vi "REQ full lifecycle.vi"(0 "endpoint":string="tcp://127.0.0.1:5555", 1 "Julia user functions script":path=path "dummy.jl", 2 "LV Client state in":T2, 5 "data to send":string="hello", 7 "ZMQ new Timeouts in":T1={"SNDTIMEO"=-1, "RCVTIMEO"=-1}, 9 "Force command":bool, 11 "error in":errorcluster, 12 "command":T3, 13 "Jl Server state in":T2) -> (3 "LV Client state out":T2, 4 "server response":string, 6 "socket out":refnum<class "zmq_socket.lvclass">, 8 "ZMQ timeouts out":cluster{"previous":T1, "current":T1}={"previous"={"SNDTIMEO"=-1, "RCVTIMEO"=-1}, "current"={"SNDTIMEO"=-1, "RCVTIMEO"=-1}}, 10 "timeout?":bool, 14 "Jl Server state out":T2, 15 "error out":errorcluster)   [LabVIEW 2018, in "LV-0mq-Julia_roundtrip-lib.lvlib"]
uses:
  LV-0mq-Julia_roundtrip-lib.lvlib
  Commands.ctl
  Server or client state.ctl
  ZMQ timeouts.ctl
  <vilib>/addons/zeromq/zmq_socket.lvclass
  <vilib>/addons/zeromq/zmq_context.lvclass
  commands LV2Jl.ctl
  expected server response.ctl
  <vilib>/addons/zeromq/socket_options.ctl
  <vilib>/Utility/error.llb/Error Cluster From Error Code.vi
  ZMQ timeouts global.vi
  <vilib>/addons/zeromq/zmq_getsocketopt_int.vi
  <vilib>/ErrorRing/Error Ring.xnode
  <vilib>/addons/zeromq/zeromq.lvlib
panel:
  out "return code":i32
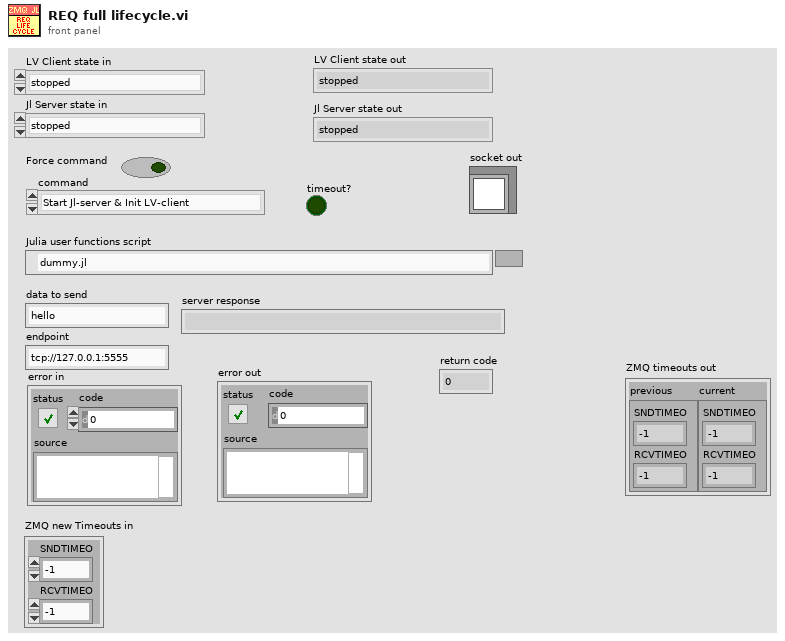
[diagram p1: front panel]
types:
  T1 = typedef "LV-0mq-Julia_roundtrip-lib.lvlib/ZMQ timeouts.ctl" = cluster{"SNDTIMEO":i32, "RCVTIMEO":i32}
  T2 = typedef "LV-0mq-Julia_roundtrip-lib.lvlib/Server or client state.ctl" = enum16{"stopped", "running", "unknown"}
  T3 = typedef "LV-0mq-Julia_roundtrip-lib.lvlib/Commands.ctl" = enum16{"Start Jl-server & Init LV-client", "Send request & Get response ", "Stop Jl-server & Cleanup LV-client", "Cleanup LV-client", "Start Jl-server", "Stop Jl-server", "Init LV-Client", "Cleanup LV-Client", "(not allowed)", "Set LV Client state", "Set Jl Server state", "set ZMQ timeout", "read ZMQ timeout", "read-out state"}
  T4 = typedef "zeromq.lvlib/socket_options.ctl" = enum8{"NONE", "ZMQ_HWM", "<2>", "ZMQ_SWAP", "ZMQ_AFFINITY", "ZMQ_IDENTITY", "ZMQ_SUBSCRIBE", "ZMQ_UNSUBSCRIBE", "ZMQ_RATE", "ZMQ_RECOVERY_IVL", "ZMQ_MCAST_LOOP", "ZMQ_SNDBUF", "ZMQ_RCVBUF", "ZMQ_RCVMORE", "ZMQ_FD", "ZMQ_EVENTS", "ZMQ_TYPE", "ZMQ_LINGER", "ZMQ_RECONNECT_IVL", "ZMQ_BACKLOG", "ZMQ_RECOVERY_IVL_MSEC", "ZMQ_RECONNECT_IVL_MAX", "ZMQ_MAXMSGSIZE", "ZMQ_SNDHWM", "ZMQ_RCVHWM", "ZMQ_MULTICAST_HOPS", "<26>", "ZMQ_RCVTIMEO", "ZMQ_SNDTIMEO", "<29>", "<30>", "ZMQ_IPV4ONLY", "ZMQ_LAST_ENDPOINT", "ZMQ_ROUTER_MANDATORY", "ZMQ_TCP_KEEPALIVE", "ZMQ_TCP_KEEPALIVE_CNT", "ZMQ_TCP_KEEPALIVE_IDLE", "ZMQ_TCP_KEEPALIVE_INTVL", "ZMQ_TCP_ACCEPT_FILTER", "ZMQ_DELAY_ATTACH_ON_CONNECT", "ZMQ_XPUB_VERBOSE"}
  T5 = typedef "expected server response.ctl" = u16
  T6 = typedef "LV-0mq-Julia_roundtrip-lib.lvlib/commands LV2Jl.ctl" = u8
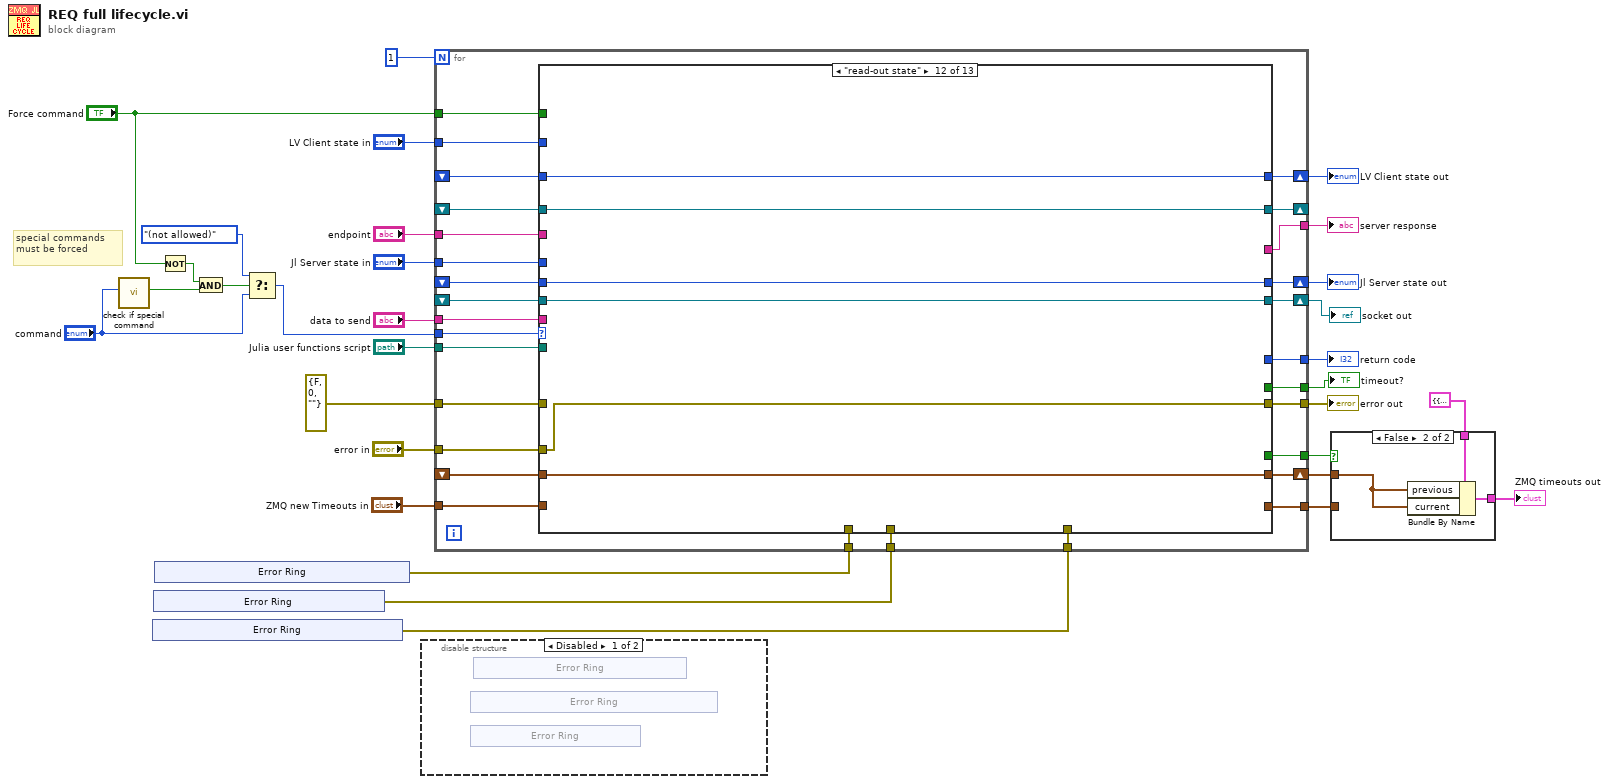
[diagram p0: block diagram]
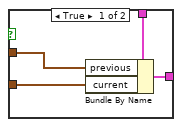
[diagram p2: hidden frame]
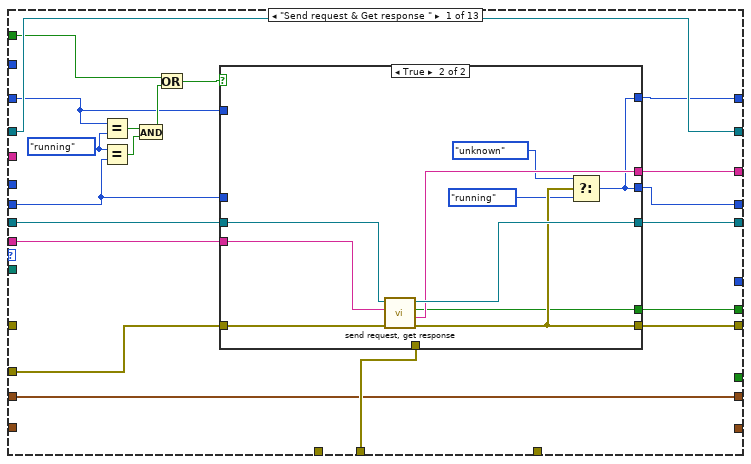
[diagram p4: hidden frame]
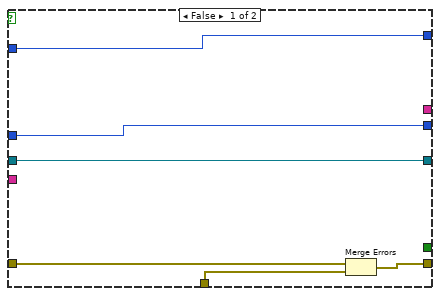
[diagram p5: hidden frame]
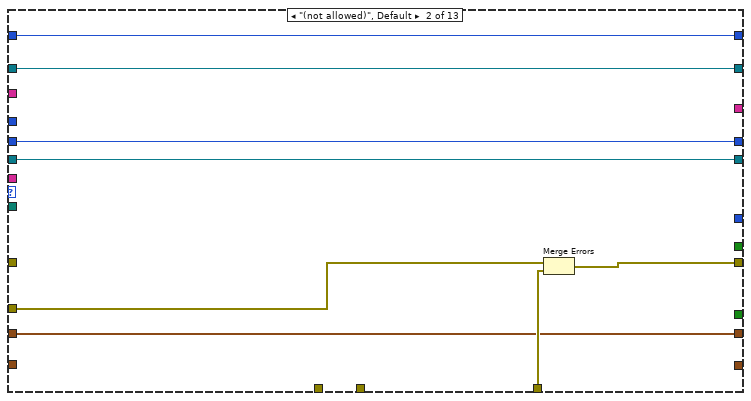
[diagram p6: hidden frame]
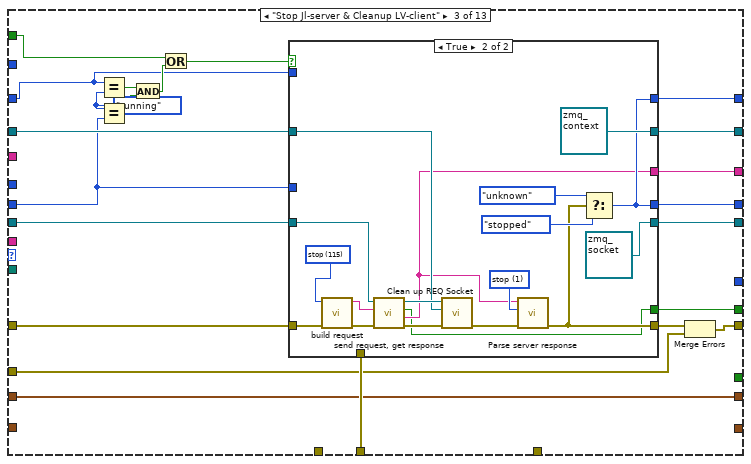
[diagram p7: hidden frame]
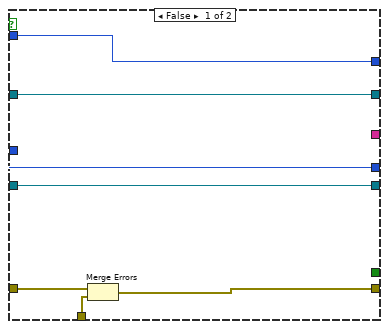
[diagram p8: hidden frame]
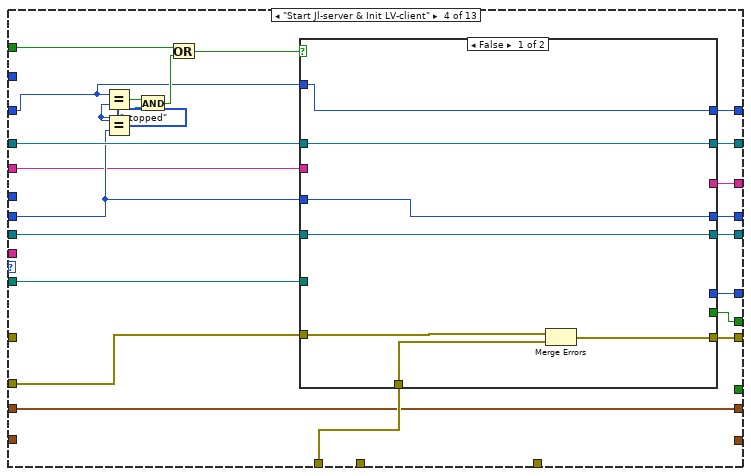
[diagram p9: hidden frame]
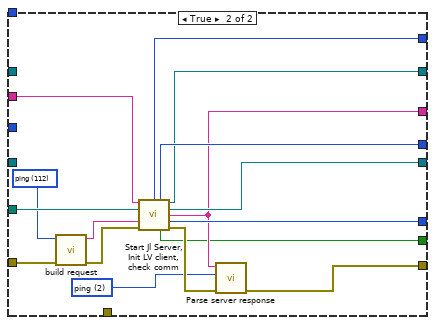
[diagram p10: hidden frame]
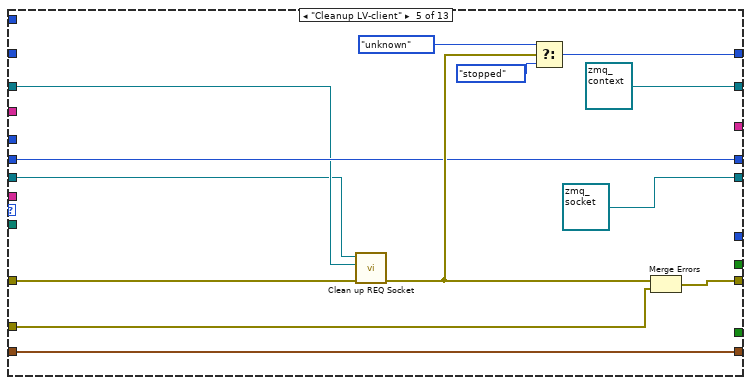
[diagram p11: hidden frame]
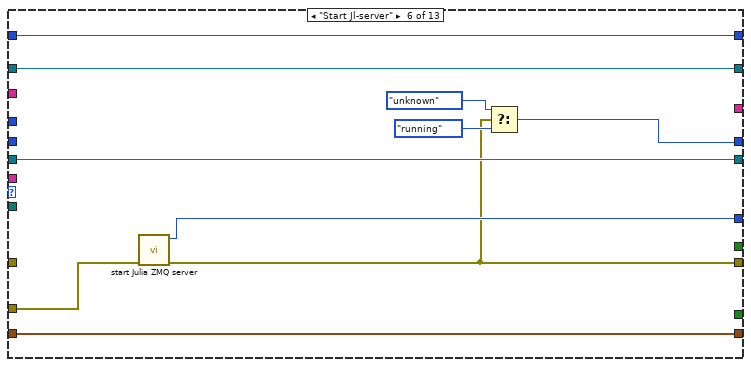
[diagram p12: hidden frame]
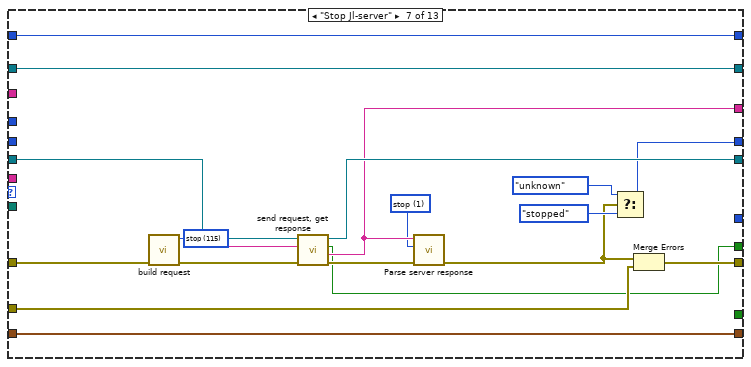
[diagram p13: hidden frame]
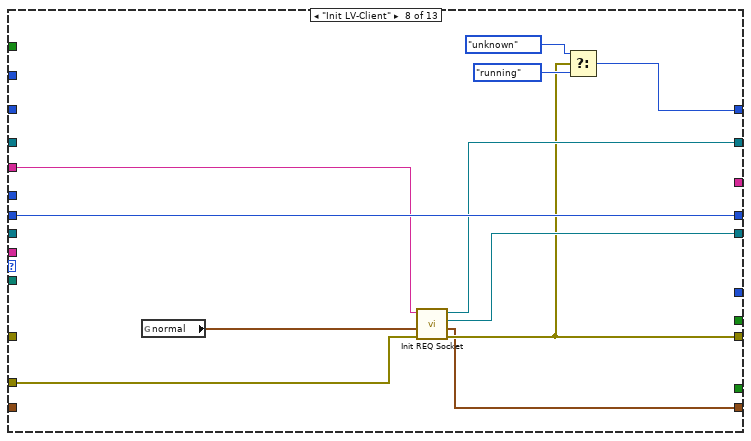
[diagram p14: hidden frame]
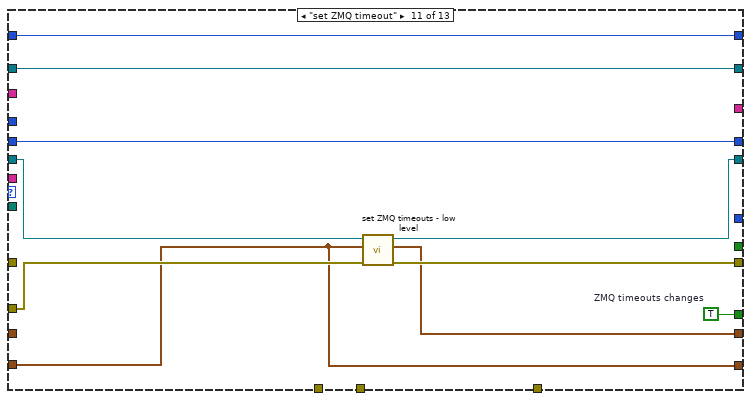
[diagram p17: hidden frame]
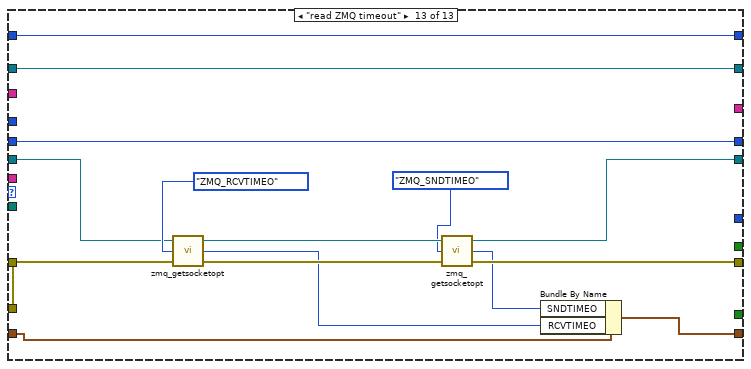
[diagram p18: hidden frame]
diagram:
  # "special commands must be forced"
  n1 = call "check if special command.vi"("command"="command") -> ("is special CMD"=w6:bool)  [unwired: 10 in]
  n2 = xnode "Error Ring"() -> ("error out"=w16:errorcluster)
  n3 = xnode "Error Ring"() -> ("error out"=w22:errorcluster)
  n4 = xnode "Error Ring"() -> ("error out"=w24:errorcluster)
  n5 = Not(x="Force command") -> (.not. x?=w20:bool)
  n6 = And(x=w20, y=w6) -> (x .and. y?=w19:bool)
  n7 = Select(t=Commands."(not allowed)" ("command"), s=w19, f="command") -> (s? t:f=w17:T3)
  n8 = disable-structure shown="Disabled" {
    frame Disabled {
      n9 = xnode "Error Ring"() -> ()  [unwired: 1 out]
      n10 = xnode "Error Ring"() -> ()  [unwired: 1 out]
      n11 = xnode "Error Ring"() -> ()  [unwired: 1 out]
    }
    frame Enabled {
    }
  }
  n12 = for {
    N: 1 -> [_]
    tunnel: [w75] -> w30
    tunnel: [w74] -> w29
    shift-right: [w73] -> _
    shift-left: _ -> [w66]
    tunnel: "endpoint" -> [w72]
    tunnel: "data to send" -> [w71]
    shift-right: [w70] -> w9
    shift-left: _ -> [w65]
    tunnel: "error in" -> [w69]
    shift-right: [w67] -> w23
    shift-left: _ -> [w68]
    tunnel: w17 -> [w64]
    tunnel: "Julia user functions script" -> [w63]
    tunnel: w24 -> [w62]
    tunnel: "Force command" -> [w61]
    shift-right: [w60] -> w15
    shift-left: _ -> [w59]
    tunnel: w22 -> [w58]
    tunnel: w16 -> [w57]
    tunnel: [w56] -> w14
    tunnel: "LV Client state in" -> [w55]
    tunnel: "Jl Server state in" -> [w54]
    tunnel: errorcluster {"status"=FALSE, "code"=0, "source"=""} ("error in") -> [w53]
    tunnel: "ZMQ new Timeouts in" -> [w52]
    tunnel: [w50] -> w8
    shift-right: [w51] -> w4
    shift-left: _ -> [w49]
    tunnel: [w48] -> w3
    tunnel: [w47] -> w2
    n13 = case shown="\"read-out state\"" w64 {
      tunnel: [w89 w118 w124 w188 w216 w227 w244 w258 w268 w274 w284 w288 w302] -> w75
      tunnel: [w90 _ w140 w177 _ _ w239 _ _ _ _ _ _] -> w74
      tunnel: [w95 w115 w135 w185 refnum<class "zmq_context.lvclass"> refnum ("zmq_context out") w232 w252 w260 w271 w276 w286 w292 w307] -> w73
      tunnel: w72 -> [_ _ _ w176 _ _ _ w257 _ _ _ _ _]
      tunnel: w71 -> [w91 _ _ _ _ _ _ _ _ _ _ _ _]
      tunnel: [w93 w113 w136 w181 refnum<class "zmq_socket.lvclass"> refnum ("zmq_socket out") w231 w251 w259 w269 w275 w281 w290 w303] -> w70
      tunnel: w69 -> [w94 w119 w123 w189 w214 w234 w242 w261 w268 w274 w283 w288 w300]
      tunnel: [w88 w114 w139 w184 w221 w228 w248 w263 w270 w273 w285 w291 w306] -> w67
      tunnel: w63 -> [_ _ _ w183 _ _ _ _ _ _ _ _ _]
      tunnel: w65 -> [w92 w113 w141 w182 w219 w231 w254 _ w269 w275 w280 w290 w295]
      tunnel: w66 -> [w95 w115 w137 w186 w220 w232 w252 _ w271 w276 w286 w292 w307]
      tunnel: w68 -> [w79 w114 w128 w180 w221 _ _ w263 w270 _ w285 w291 w306]
      tunnel: w62 -> [_ _ _ w187 _ _ _ _ _ _ _ _ _]
      tunnel: w61 -> [w82 _ w129 w178 _ _ _ _ _ _ _ _ _]
      tunnel: [w87 w116 w127 w175 w222 w235 w253 w262 w267 w277 w287 w293 w308] -> w60
      tunnel: w59 -> [w80 w116 w125 w170 _ w235 w253 _ _ w277 w287 w293 w308]
      tunnel: w58 -> [w78 _ w126 _ _ _ _ _ _ _ _ _ _]
      tunnel: w57 -> [_ w117 _ _ _ _ _ _ _ _ _ _ _]
      tunnel: [_ _ _ w169 _ w233 _ _ _ _ _ _ _] -> w56
      tunnel: w55 -> [_ _ _ _ _ _ _ _ w267 _ _ _ _]
      tunnel: w54 -> [_ _ _ _ _ _ _ _ _ w273 _ _ _]
      tunnel: w53 -> [_ _ w122 _ w215 _ w243 _ _ _ _ _ _]
      tunnel: w52 -> [_ _ _ _ _ _ _ _ _ _ w278 _ _]
      tunnel: [w76 w112 w120 w167 w213 w226 w236 w256 w266 w272 w282 w289 w298] -> w51
      tunnel: [w77 _ w121 w168 _ _ w237 _ _ _ _ _ _] -> w50
      tunnel: w49 -> [w76 w112 w120 w167 w213 w226 w236 _ w266 w272 _ w289 w294]
      tunnel: [_ _ _ _ _ _ _ _ _ _ w279 _ _] -> w47
      tunnel: [_ _ _ _ _ _ _ _ _ _ w278 _ _] -> w48
      frame "Send request & Get response " {
        w85 = Server_or_client_state."running" ("Server state")
        n14 = Equal?(x=w80, y=w85) -> (x = y?=w83:bool)
        n15 = Equal?(x=w85, y=w79) -> (x = y?=w86:bool)
        n16 = And(x=w83, y=w86) -> (x .and. y?=w84:bool)
        n17 = Or(x=w82, y=w84) -> (x .or. y?=w81:bool)
        n18 = case shown="True" w81 {
          tunnel: w94 -> [w98 w111]
          tunnel: [w99 w110] -> w93
          tunnel: w92 -> [w99 w109]
          tunnel: w91 -> [_ w108]
          tunnel: [_ w107] -> w90
          tunnel: [w97 w105] -> w89
          tunnel: [w100 w104] -> w88
          tunnel: w79 -> [w100 _]
          tunnel: [w101 w104] -> w87
          tunnel: w80 -> [w101 _]
          tunnel: w78 -> [w96 _]
          tunnel: [_ w102] -> w77
          frame False {
            n19 = Merge Errors(w98, w96) -> (w97:errorcluster)
          }
          frame True {
            n20 = call "send request, get response.vi"("error in (no error)"=w111, "request"=w108, "zmq_socket in"=w109) -> ("error out"=w105:errorcluster, "response"=w107:string, "timeout?"=w102:bool, "zmq_socket out"=w110:refnum<class "zmq_socket.lvclass">)  [unwired: 4 in, 1 out]
            n21 = Select(t=Server_or_client_state."unknown" ("Server state"), s=w105, f=Server_or_client_state."running" ("Server state")) -> (s? t:f=w104:T2)
          }
        }
      }
      frame "(not allowed)", Default {
        n22 = Merge Errors(w119, w117) -> (w118:errorcluster)
      }
      frame "Stop Jl-server & Cleanup LV-client" {
        w133 = Server_or_client_state."running" ("Server state")
        n23 = Equal?(x=w125, y=w133) -> (x = y?=w131:bool)
        n24 = Equal?(x=w133, y=w128) -> (x = y?=w134:bool)
        n25 = And(x=w131, y=w134) -> (x .and. y?=w132:bool)
        n26 = Or(x=w129, y=w132) -> (x .or. y?=w130:bool)
        n27 = case shown="True" w130 {
          tunnel: w122 -> [w144 w157]
          tunnel: w141 -> [w146 w166]
          tunnel: [_ w150] -> w140
          tunnel: [w148 w159] -> w139
          tunnel: [w143 w151] -> w138
          tunnel: w137 -> [w145 w154]
          tunnel: [w146 refnum<class "zmq_socket.lvclass"> refnum ("zmq_socket out")] -> w136
          tunnel: [w145 refnum<class "zmq_context.lvclass"> refnum ("zmq_context out")] -> w135
          tunnel: w128 -> [w148 _]
          tunnel: [w147 w159] -> w127
          tunnel: w125 -> [w147 _]
          tunnel: w126 -> [w142 _]
          tunnel: [_ w149] -> w121
          frame False {
            n28 = Merge Errors(w144, w142) -> (w143:errorcluster)
          }
          frame True {
            w153 = T5 1 items=["detailed response", "stop", "ping"] ("expected response")
            w156 = T6 115 items=["call function"=99, "ping"=112, "stop"=115] ("Command")
            n29 = call "build request.vi"("error in (no error)"=w157, "Command"=w156) -> ("error out"=w158:errorcluster, "REQ string"=w155:string)  [unwired: 8 in]
            n30 = call "send request, get response.vi"("error in (no error)"=w158, "request"=w155, "zmq_socket in"=w166) -> ("error out"=w164:errorcluster, "response"=w150:string, "timeout?"=w149:bool, "zmq_socket out"=w162:refnum<class "zmq_socket.lvclass">)  [unwired: 4 in, 1 out]
            n31 = call "Clean up REQ Socket.vi"("error in (no error)"=w164, "zmq_context in"=w154, "zmq_socket in"=w162) -> ("error out"=w152:errorcluster)  [unwired: 8 in]
            n32 = call "Parse server response.vi"("error in (no error)"=w152, "expected response"=w153, "server response in"=w150) -> ("error out"=w151:errorcluster)  [unwired: 2 in, 6 out]
            n33 = Select(t=Server_or_client_state."unknown" ("Server state"), s=w151, f=Server_or_client_state."stopped") -> (s? t:f=w159:T2)
          }
        }
        n34 = Merge Errors(w138, w123) -> (w124:errorcluster)
      }
      frame "Start Jl-server & Init LV-client" {
        w173 = Server_or_client_state."stopped" ("Server state")
        n35 = Equal?(x=w170, y=w173) -> (x = y?=w171:bool)
        n36 = Equal?(x=w173, y=w180) -> (x = y?=w174:bool)
        n37 = And(x=w171, y=w174) -> (x .and. y?=w172:bool)
        n38 = Or(x=w178, y=w172) -> (x .or. y?=w179:bool)
        n39 = case shown="False" w179 {
          tunnel: w189 -> [w196 w204]
          tunnel: [w195 w200] -> w188
          tunnel: w187 -> [w194 _]
          tunnel: [w193 w209] -> w185
          tunnel: w186 -> [w193 _]
          tunnel: [w192 w210] -> w184
          tunnel: w180 -> [w192 _]
          tunnel: w183 -> [_ w212]
          tunnel: [w191 w208] -> w181
          tunnel: w182 -> [w191 _]
          tunnel: [_ w199] -> w177
          tunnel: w176 -> [_ w211]
          tunnel: [w190 w207] -> w175
          tunnel: w170 -> [w190 _]
          tunnel: [_ w206] -> w169
          tunnel: [_ w197] -> w168
          frame False {
            n40 = Merge Errors(w196, w194) -> (w195:errorcluster)
          }
          frame True {
            w198 = T5 2 items=["detailed response", "stop", "ping"] ("expected response")
            w203 = T6 112 items=["call function"=99, "ping"=112, "stop"=115] ("Command")
            n41 = call "build request.vi"("error in (no error)"=w204, "Command"=w203) -> ("error out"=w205:errorcluster, "REQ string"=w202:string)  [unwired: 8 in]
            n42 = call "Start Jl Server, Init LV client, check comm.vi"("endpoint"=w211, "Julia user functions script"=w212, "request"=w202, "error in (no error)"=w205) -> ("LV client state"=w207:T2, "JL server state"=w210:T2, "zmq_context out"=w209:refnum<class "zmq_context.lvclass">, "zmq_socket out"=w208:refnum<class "zmq_socket.lvclass">, "response"=w199:string, "script return code (0)"=w206:i32, "timeout?"=w197:bool, "error out"=w201:errorcluster)  [unwired: 4 in]
            n43 = call "Parse server response.vi"("error in (no error)"=w201, "expected response"=w198, "server response in"=w199) -> ("error out"=w200:errorcluster)  [unwired: 2 in, 6 out]
          }
        }
      }
      frame "Cleanup LV-client" {
        n44 = call "Clean up REQ Socket.vi"("error in (no error)"=w215, "zmq_context in"=w220, "zmq_socket in"=w219) -> ("error out"=w223:errorcluster)  [unwired: 8 in]
        n45 = Select(t=Server_or_client_state."unknown" ("Server state"), s=w223, f=Server_or_client_state."stopped") -> (s? t:f=w222:T2)
        n46 = Merge Errors(w223, w214) -> (w216:errorcluster)
      }
      frame "Start Jl-server" {
        n47 = call "start Julia ZMQ server.vi"("error in (no error)"=w234) -> ("error out"=w227:errorcluster, "return code"=w233:i32)  [unwired: 9 in]
        n48 = Select(t=Server_or_client_state."unknown" ("Server state"), s=w227, f=Server_or_client_state."running") -> (s? t:f=w228:T2)
      }
      frame "Stop Jl-server" {
        w238 = T5 1 items=["detailed response", "stop", "ping"] ("expected response")
        w246 = T6 115 items=["call function"=99, "ping"=112, "stop"=115] ("Command")
        n49 = call "build request.vi"("error in (no error)"=w243, "Command"=w246) -> ("error out"=w247:errorcluster, "REQ string"=w245:string)  [unwired: 8 in]
        n50 = call "send request, get response.vi"("error in (no error)"=w247, "request"=w245, "zmq_socket in"=w254) -> ("error out"=w241:errorcluster, "response"=w239:string, "timeout?"=w237:bool, "zmq_socket out"=w251:refnum<class "zmq_socket.lvclass">)  [unwired: 4 in, 1 out]
        n51 = call "Parse server response.vi"("error in (no error)"=w241, "expected response"=w238, "server response in"=w239) -> ("error out"=w240:errorcluster)  [unwired: 2 in, 6 out]
        n52 = Select(t=Server_or_client_state."unknown" ("Server state"), s=w240, f=Server_or_client_state."stopped") -> (s? t:f=w248:T2)
        n53 = Merge Errors(w240, w242) -> (w244:errorcluster)
      }
      frame "Init LV-Client" {
        n54 = global read "ZMQ timeouts global.vi" "normal"() -> (w255:T1)
        n55 = call "Init REQ Socket.vi"("error in (no error)"=w261, "ZMQ new Timeouts in"=w255, "endpoint"=w257) -> ("error out"=w258:errorcluster, "ZMQ new Timeouts out"=w256:T1, "socket out"=w259:refnum<class "zmq_socket.lvclass">, "zmq_context out"=w260:refnum<class "zmq_context.lvclass">)  [unwired: 5 in]
        n56 = Select(t=Server_or_client_state."unknown" ("Server state"), s=w258, f=Server_or_client_state."running") -> (s? t:f=w262:T2)
      }
      frame "Set LV Client state" {
      }
      frame "Set Jl Server state" {
      }
      frame "set ZMQ timeout" {
        w279 = TRUE  # ZMQ timeouts changes
        n57 = call "set ZMQ timeouts - low level.vi"("error in (no error)"=w283, "ZMQ new Timeouts in"=w278, "zmq_socket in"=w280) -> ("error out"=w284:errorcluster, "ZMQ new Timeouts out"=w282:T1, "zmq_socket out"=w281:refnum<class "zmq_socket.lvclass">)  [unwired: 6 in]
      }
      frame "read-out state" {
      }
      frame "read ZMQ timeout" {
        n58 = call-poly <vilib>:"zmq_getsocketopt.vi"("error in"=w300, "option"=socket_options."ZMQ_RCVTIMEO", "socket in"=w295) -> ("error out"=w305:errorcluster, "value"=w297:i32, "socket out"=w304:refnum<class "zmq_socket.lvclass">)
        n59 = call-poly <vilib>:"zmq_getsocketopt.vi"("error in"=w305, "option"=socket_options."ZMQ_SNDTIMEO", "socket in"=w304) -> ("error out"=w302:errorcluster, "value"=w296:i32, "socket out"=w303:refnum<class "zmq_socket.lvclass">)
        n60 = Bundle By Name(cluster=w294, "SNDTIMEO"=w296, "RCVTIMEO"=w297) -> (w298:T1)
      }
    }
  }
  "error out" <- w30
  "server response" <- w29
  "Jl Server state out" <- w23
  "LV Client state out" <- w15
  "return code" <- w14
  "socket out" <- w9
  "timeout?" <- w8
  n61 = case shown="False" w2 {
    tunnel: [w312 w315] -> w5
    tunnel: w4 -> [w311 w313]
    tunnel: w3 -> [w310 _]
    tunnel: cluster{"previous":T1, "current":T1} {"previous"={"SNDTIMEO"=-1, "RCVTIMEO"=-1}, "current"={"SNDTIMEO"=-1, "RCVTIMEO"=-1}} ("ZMQ timeouts out") -> [w309 w314]
    frame True {
      n62 = Bundle By Name(cluster=w309, "previous"=w311, "current"=w310) -> (w312:cluster{"previous":T1, "current":T1})
    }
    frame False {
      n63 = Bundle By Name(cluster=w314, "previous"=w313, "current"=w313) -> (w315:cluster{"previous":T1, "current":T1})
    }
  }
  "ZMQ timeouts out" <- w5
